vi "ExTestPutF32.vi"() -> ()   [LabVIEW 2010]
panel:
  out "Image Display 2":sgl[][](graph)
  out "error out":errorcluster
  in  "error in (no error)":errorcluster
  out "Image Display":i32[][](graph)
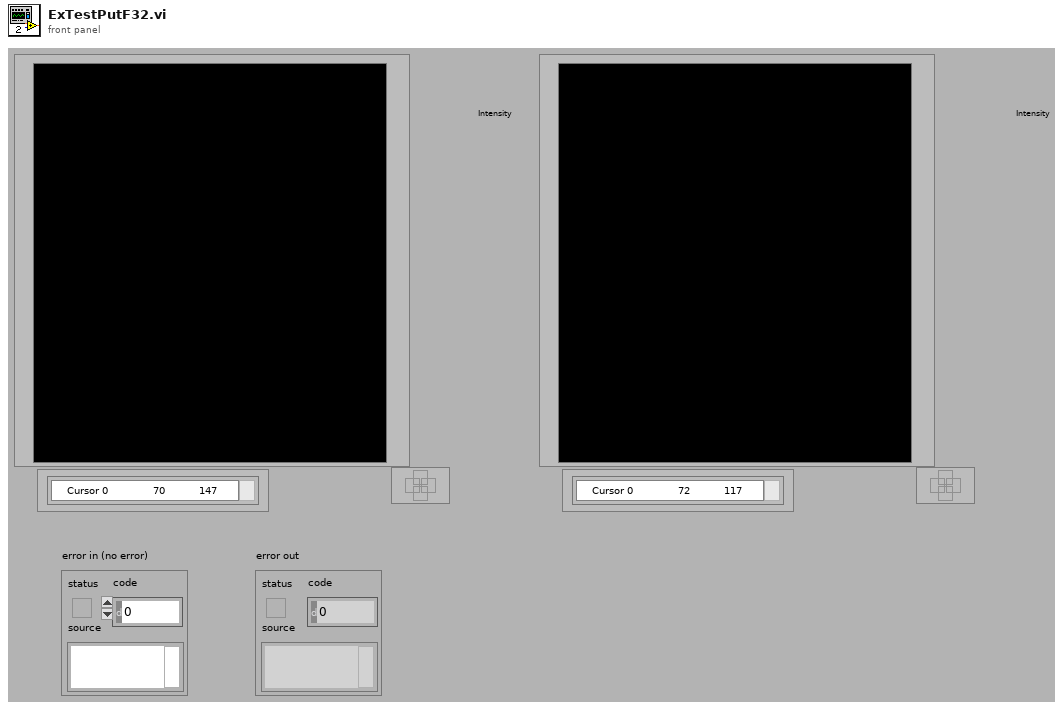
[diagram p1: front panel]
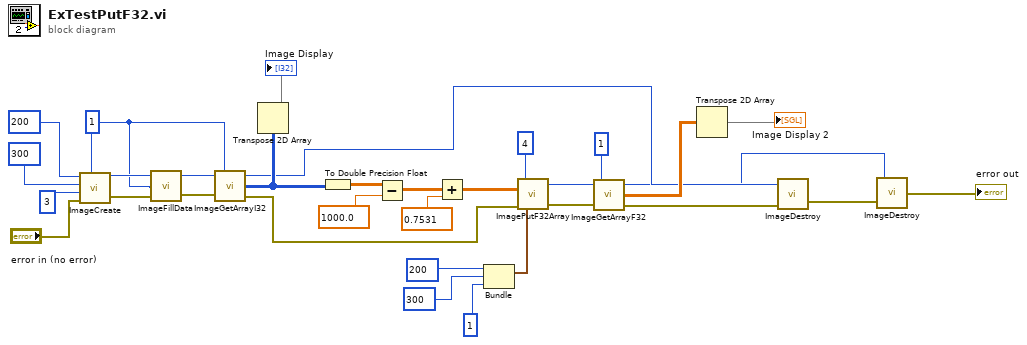
[diagram p0: block diagram]
diagram:
  w23 = 1
  n1 = call <userlib>:"ImageCreate.vi"("X dimension"=200, "Y dimension"=300, "Data Type"=3, "error in"="error in (no error)", "Number Of Frames"=w23) -> ("Image Handle"=w27:u32, "error out"=w28:errorcluster)
  n2 = call <userlib>:"ImageFillData.vi"("error in"=w28, "Type of Test"=w23, "Image Handle"=w27) -> ("error out"=w26:errorcluster, "Image Handle"=w25:u32)
  n3 = call <userlib>:"ImageGetArrayI32.vi"("error in"=w26, "Z position"=w23, "Image Handle"=w25) -> ("error out"=w15:errorcluster, "Array int 32"=w21:i32[][], "Image Handle"=w9:u32)
  n4 = Transpose 2D Array(2D array=w21) -> (transposed array=→"Image Display":i32[][])
  n5 = To Double Precision Float(number=w21) -> (double precision float=w20:dbl[][])
  n6 = Subtract(x=w20, y=1000.0) -> (x-y=w18:dbl[][])
  n7 = Add(x=w18, y=0.7531) -> (x+y=w16:dbl[][])
  n8 = Bundle(200, 300, 1) -> (w4:cluster{i32, i32, i32})  [unwired: 1 in]
  n9 = call <userlib>:"ImagePutF32Array.vi"("error in (no error)"=w15, "Image dimensions"=w4, "Image Data"=w16, "Data Type to store as"=4) -> ("error out"=w14:errorcluster, "Image Handle"=w13:u32)
  n10 = call <userlib>:"ImageGetArrayF32.vi"("error in"=w14, "Z position"=1, "Image Handle"=w13) -> ("error out"=w8:errorcluster, "Array Float 32"=w11:sgl[][], "Image Handle"=w6:u32)
  n11 = Transpose 2D Array(2D array=w11) -> (transposed array=→"Image Display 2":sgl[][])
  n12 = call <userlib>:"ImageDestroy.vi"("error in"=w8, "Data handle"=w9) -> ("error out"=w7:errorcluster)
  n13 = call <userlib>:"ImageDestroy.vi"("error in"=w7, "Data handle"=w6) -> ("error out"=→"error out":errorcluster)
